vi "display.vi"(8 "error in (no error)":errorcluster, 11 "DL090216Display in":refnum<class "DisplayDL090216.lvclass">) -> (0 "error out":errorcluster, 3 "DL090216Display out":refnum<class "DisplayDL090216.lvclass">)   [LabVIEW 2010, in "DisplayDL090216.lvclass"]
uses:
  DisplayDL090216.lvclass
  DisplayDL090216.lvclass/DisplayDL090216.ctl
  common/classes/Image/Image/Image.lvclass
  ImageProcessor/ImageProcessorDL090216RangeOffset/ImageProcessorDL090216RangeOffset/ImageProcessorDL090216RangeOffset.lvclass
  individual_channel_cluster.ctl
  <vilib>/vision/Image Controls.llb/IMAQ Image.ctl
  common/classes/ErrorController/ErrorController/class_data.vi
  common/classes/ErrorController/ErrorController/ErrorController.lvclass
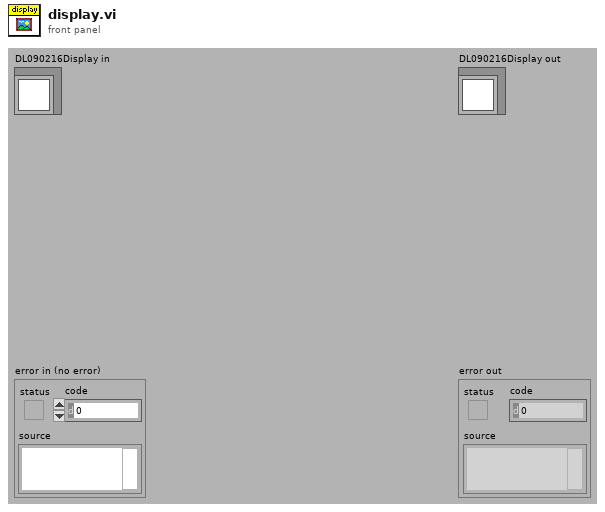
[diagram p1: front panel]
types:
  T1 = typedef "DisplayDL090216.lvclass/individual_channel_cluster.ctl" = cluster{"Image":T2, "histogram out":cluster{i32, u32}[], "button:color scale":bool, "button:set as main image":bool}
  T2 = typedef "IMAQ Image.ctl" = refnum<image>
  T3 = typedef "Image.lvclass/colour_enum.ctl" = enum16{"none", "red", "green", "blue", "grey scale", "custom"}
  T4 = cluster{"channel histogram":cluster{i32, u32}[]}[]
  T5 = typedef "Image.lvclass/unit.ctl" = enum16{"um", "s"}
  T6 = typedef "range_offset_cluster.ctl" = cluster{"range":dbl, "offset":dbl}
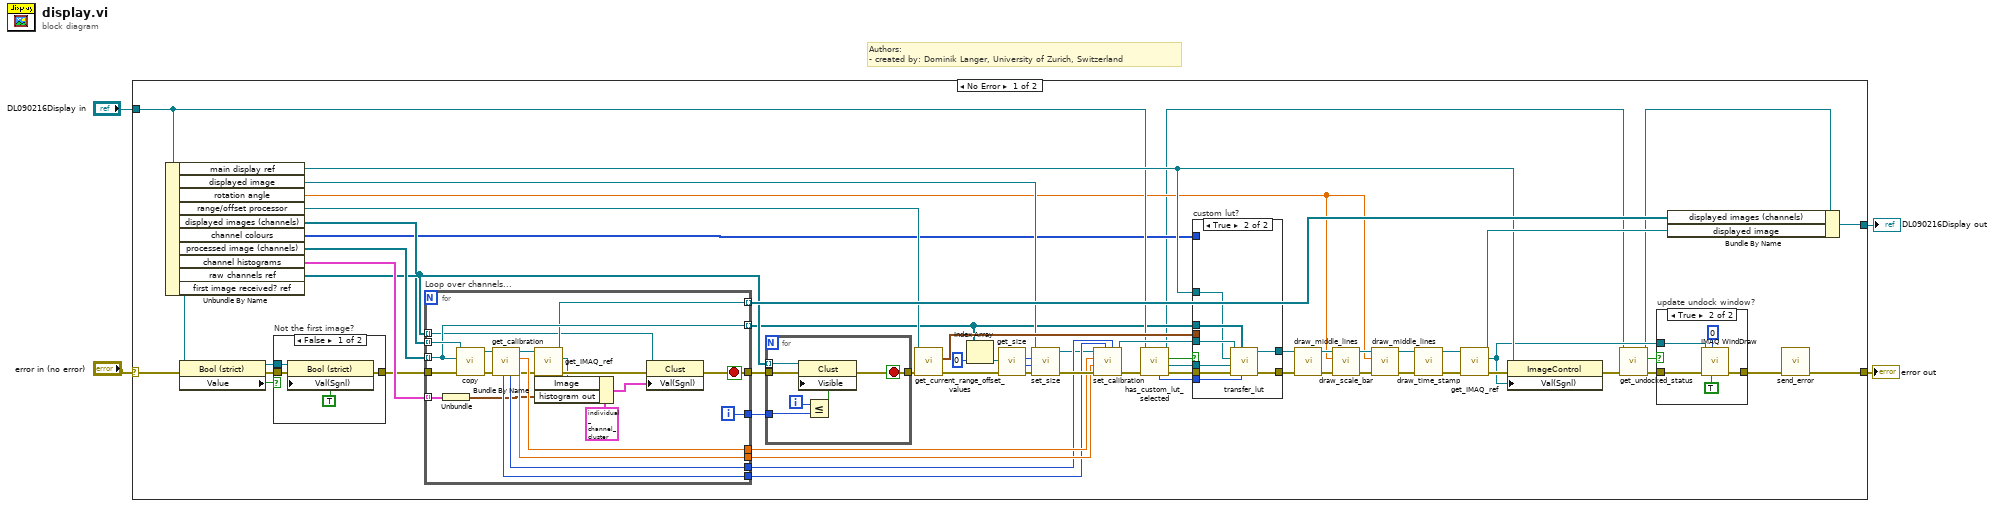
[diagram p0: block diagram]
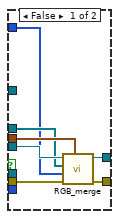
[diagram p3: hidden frame]
diagram:
  # "Authors: \n- created by: Dominik Langer, University of Zurich, Switzerland"
  n1 = case shown="No Error" "error in (no error)" {
    selector: "error in (no error)" -> [w27 w120]
    tunnel: [w22 w120] -> w3
    tunnel: [w29 w119] -> w1
    tunnel: "DL090216Display in" -> [w20 w119]
    frame No Error {
      n2 = Unbundle By Name(w20) -> ("main display ref"=w21:refnum<vi>, "displayed image"=w46:refnum<class "Image.lvclass">, "rotation angle"=w16:dbl[unit], "range/offset processor"=w52:refnum<class "ImageProcessorDL090216RangeOffset.lvclass">, "displayed images (channels)"=w31:refnum<class "Image.lvclass">[], "channel colours"=w15:T3[], "processed image (channels)"=w58:refnum<class "Image.lvclass">[], "channel histograms"=w35:T4, "raw channels ref"=w32:refnum<vi>[], "first image received? ref"=w28:refnum<vi>)
      n3 = property class="Bool (strict)"(reference=w28, error in=w27) -> (reference out=w26:refnum<vi>, error out=w25:errorcluster, "Value"=w24:bool)
      n4 = case "Not the first image?" shown="False" w24 {
        tunnel: w25 -> [w90 w91]
        tunnel: [w89 w91] -> w23
        tunnel: w26 -> [w88 _]
        frame False {
          n5 = property class="Bool (strict)"(reference=w88, error in=w90, "Val(Sgnl)"=TRUE) -> (error out=w89:errorcluster)  [unwired: 1 out]
        }
        frame True {
        }
      }
      n6 = for "Loop over channels..." {
        tunnel: w58 -> [w111] mode=indexing
        tunnel: [w111] -> w8 mode=indexing
        tunnel: w31 -> [w118] mode=indexing
        tunnel: [w109] -> w57 mode=indexing
        tunnel: [w115] -> w54
        tunnel: [w114] -> w53
        tunnel: [w113] -> w48
        tunnel: [w112] -> w49
        tunnel: w35 -> [w106] mode=indexing
        tunnel: w32 -> [w102] mode=indexing
        tunnel: [w103] -> w34
        tunnel: [w101] -> w30
        tunnel: w23 -> [w98]
        i -> [w101]
        stop <- w103 stop-if-true
        n7 = Unbundle(w106) -> ("channel histogram"=w105:cluster{i32, u32}[])
        n8 = call "copy.vi"("error in (no error)"=w98, "image to copy (source)"=w111, "Image in (target)"=w118) -> ("error out"=w116:errorcluster, "Image out"=w117:refnum<class "Image.lvclass">)  [unwired: 7 out]
        n9 = call "get_calibration.vi"("error in (no error)"=w116, "Image.lvclass in"=w117) -> ("error out"=w108:errorcluster, "y"=w114:dbl, "x"=w115:dbl, "Image.lvclass out"=w107:refnum<class "Image.lvclass">, "y unit"=w113:T5, "x unit"=w112:T5)  [unwired: 4 out]
        n10 = call-dynamic "get_IMAQ_ref.vi"("error in (no error)"=w108, "Image.lvclass in"=w107) -> ("error out"=w104:errorcluster, "Image"=w100:T2, "Image.lvclass out"=w109:refnum<class "Image.lvclass">)  [unwired: 7 out]
        n11 = Bundle By Name(cluster=T1 {"Image"=refnum, "histogram out"=[], "button:color scale"=FALSE, "button:set as main image"=FALSE} ("individual channel"), "Image"=w100, "histogram out"=w105) -> (w99:T1)
        n12 = property class="Clust"(reference=w102, error in=w104, "Val(Sgnl)"=w99) -> (error out=w103:errorcluster)  [unwired: 1 out]
      }
      n13 = for {
        tunnel: w34 -> [w97]
        tunnel: [w96] -> w33
        tunnel: w32 -> [w95] mode=indexing
        tunnel: w30 -> [w92]
        i -> [w93]
        stop <- w96 stop-if-true
        n14 = Less Or Equal?(x=w93, y=w92) -> (x <= y?=w94:bool)
        n15 = property class="Clust"(reference=w95, error in=w97, "Visible"=w94) -> (error out=w96:errorcluster)  [unwired: 1 out]
      }
      n16 = call-dynamic "get_current_range_offset_values.vi"("error in (no error)"=w33, "DL090216RangeOffsetImageProcessor in"=w52) -> ("error out"=w51:errorcluster, "range offset values (channels)"=w50:T6[])  [unwired: 8 out]
      n17 = Index Array(array=w8, index=0) -> (element=w62:refnum<class "Image.lvclass">)
      n18 = call-dynamic "get_size.vi"("error in (no error)"=w51, "Image in"=w62) -> ("error out"=w59:errorcluster, "y resolution"=w60:i32, "x resolution"=w61:i32)  [unwired: 7 out]
      n19 = call-dynamic "set_size.vi"("error in (no error)"=w59, "y"=w60, "x"=w61, "Image in"=w46) -> ("error out"=w56:errorcluster, "Image out"=w47:refnum<class "Image.lvclass">)  [unwired: 6 out]
      n20 = call "set_calibration.vi"("y unit"=w48, "x unit"=w49, "error in (no error)"=w56, "y"=w53, "x"=w54, "Image in"=w47) -> ("error out"=w19:errorcluster, "Image out"=w55:refnum<class "Image.lvclass">)  [unwired: 4 out]
      n21 = call-dynamic "has_custom_lut_selected.vi"("error in (no error)"=w19, "DisplayDL090216 in"=w20) -> ("error out"=w18:errorcluster, "channel"=w14:refnum<vi>, "has custom selected?"=w17:bool, "DisplayDL090216 out"=w7:refnum<class "DisplayDL090216.lvclass">, "index of element"=w13:i32)  [unwired: 5 in]
      n22 = case "custom lut?" shown="True" w17 {
        tunnel: w55 -> [w78 w86]
        tunnel: w18 -> [w77 w84]
        tunnel: w50 -> [w76 _]
        tunnel: [w75 w83] -> w45
        tunnel: [w74 w85] -> w44
        tunnel: w8 -> [w73 w82]
        tunnel: w15 -> [w72 _]
        tunnel: w21 -> [_ w81]
        tunnel: w14 -> [_ w80]
        tunnel: w13 -> [_ w79]
        frame False {
          n23 = call-dynamic "RGB_merge.vi"("offset and range"=w76, "error in (no error)"=w77, "colours"=w72, "images"=w73, "Image in"=w78) -> ("error out"=w75:errorcluster, "Image out"=w74:refnum<class "Image.lvclass">)  [unwired: 5 out]
        }
        frame True {
          n24 = call-dynamic "transfer_lut.vi"("index of element"=w79, "images"=w82, "error in (no error)"=w84, "source"=w80, "destination"=w81, "Image in"=w86) -> ("error out"=w83:errorcluster, "Image out"=w85:refnum<class "Image.lvclass">)  [unwired: 4 in]
        }
      }
      n25 = call "draw_middle_lines.vi"("error in (no error)"=w45, "Image in"=w44) -> ("error out"=w43:errorcluster, "Image out"=w42:refnum<class "Image.lvclass">)  [unwired: 1 in, 7 out]
      n26 = call "draw_scale_bar.vi"("error in (no error)"=w43, "angle"=w16, "Image in"=w42) -> ("error out"=w41:errorcluster, "Image out"=w40:refnum<class "Image.lvclass">)  [unwired: 2 in, 5 out]
      n27 = call "draw_middle_lines.vi"("error in (no error)"=w41, "rotation angle"=w16, "Image in"=w40) -> ("error out"=w39:errorcluster, "Image out"=w38:refnum<class "Image.lvclass">)  [unwired: 7 in]
      n28 = call "draw_time_stamp.vi"("error in (no error)"=w39, "Image in"=w38) -> ("error out"=w36:errorcluster, "Image out"=w37:refnum<class "Image.lvclass">)  [unwired: 8 in]
      n29 = call-dynamic "get_IMAQ_ref.vi"("error in (no error)"=w36, "Image.lvclass in"=w37) -> ("error out"=w64:errorcluster, "Image"=w9:T2, "Image.lvclass out"=w65:refnum<class "Image.lvclass">)  [unwired: 7 out]
      n30 = property class="ImageControl"(reference=w21, error in=w64, "Val(Sgnl)"=w9) -> (error out=w12:errorcluster)  [unwired: 1 out]
      n31 = call-dynamic "get_undocked_status.vi"("error in (no error)"=w12, "DisplayDL090216 in"=w7) -> ("error out"=w10:errorcluster, "has undocked window?"=w11:bool, "DisplayDL090216 out"=w6:refnum<class "DisplayDL090216.lvclass">)  [unwired: 7 in]
      n32 = case "update undock window?" shown="True" w11 {
        tunnel: [w66 w70] -> w5
        tunnel: w10 -> [w66 w71]
        tunnel: w9 -> [_ w68]
        frame False {
        }
        frame True {
          n33 = call "IMAQ WindDraw"("Resize to Image Size? (Y)"=TRUE, "Window Number (0...15)"=0, "error in (no error)"=w71, "Image"=w68) -> ("error out"=w70:errorcluster)  [unwired: 6 in, 1 out]
        }
      }
      n34 = Bundle By Name(cluster=w6, "displayed images (channels)"=w57, "displayed image"=w65) -> (w29:refnum<class "DisplayDL090216.lvclass">)
      n35 = call "send_error.vi"("error in (no error)"=w5) -> ("error out"=w22:errorcluster)  [unwired: 10 in]
    }
    frame Error {
    }
  }
  "error out" <- w3
  "DL090216Display out" <- w1
